vi "degree-to-rad (SubVI).vi"(11 "oblique angle":dbl) -> (3 "Numeric":dbl)   [LabVIEW 2024]
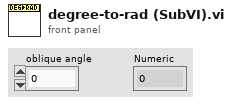
[diagram p1: front panel]
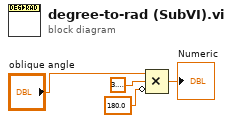
[diagram p0: block diagram]
diagram:
  n1 = Compound Arithmetic op=MULTIPLY("oblique angle", 3.141592653589793, invert 180.0 ("value")) -> (→"Numeric":dbl)
